vi "Data to Label and Time Tag and Buffer Report Word.vi"(11 "Rx data":T1) -> (2 "buffer report word":u32 format="%032b", 3 "data word":u32 format="%032b", 5 "time stamp":timestamp)   [LabVIEW 2020, in "AIM ARINC 429 Hardware API.lvlib"]
uses:
  AIM ARINC 429 Hardware API.lvlib
  <instrlib>/AIM GmbH/ARINC-429/Controls/rx_stack_entry.ctl
  <instrlib>/AIM GmbH/ARINC-429/AIM429LV.lvlib
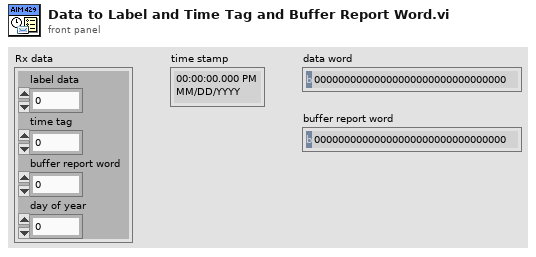
[diagram p1: front panel]
types:
  T1 = typedef "AIM429LV.lvlib/rx_stack_entry.ctl" = cluster{"label data":u32, "time tag":u32, "buffer report word":u32, "day of year":u32}
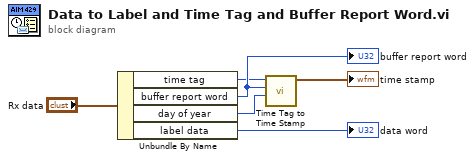
[diagram p0: block diagram]
diagram:
  n1 = Unbundle By Name("Rx data") -> ("time tag"=w2:u32, "buffer report word"=w4:u32, "day of year"=w1:u32, "label data"=→"data word":u32)
  "buffer report word" <- w4
  n2 = call "Time Tag to Time Stamp.vi"("day of year"=w1, "buffer report word"=w4, "time tag"=w2) -> ("time stamp"=→"time stamp":timestamp)  [unwired: 7 in, 1 out]
